vi "SettingButton_MenuSelect by Path.vi"(8 "error in (no error)":errorcluster caption="错误输入（无错误）", 9 "QName":string, 10 "MenuPath":string, 11 "PCM PanelSplit 输入":refnum<class "PCM PanelSplit.lvclass"> caption="DNL_LabVIEW Object in") -> (0 "error out":errorcluster caption="错误输出", 3 "PCM PanelSplit 输出":refnum<class "PCM PanelSplit.lvclass"> caption="DNL_LabVIEW Object out")   [LabVIEW 2016, in "PCM PanelSplit.lvclass"]
uses:
  PCM PanelSplit.lvclass
  Display Mode.ctl
  <vilib>/Analysis/4window.llb/windowTd.ctl
  PanelSplitToolkit/QueueManager.llb/Insert.vi
  <vilib>/Analysis/NI_AALPro.lvlib
panel:
  in  "window":T1=1 caption="窗" items=["Rectangle"=0, "Hanning"=1, "Hamming"=2, "Blackman-Harris"=3, "Exact Blackman"=4, "Blackman"=5, "Flat Top"=6, "4 Term B-Harris "=7, "7 Term B-Harris"=8, "Low Sidelobe"=9, "Blackman Nuttall"=11, "Triangle"=30, "Bartlett-Hanning"=31, "Bohman"=32, "Parzen"=33, "Welch"=34, "Kaiser"=60, "Dolph-Chebyshev"=61, "Gaussian"=62]
  in  "Display Mode":T2
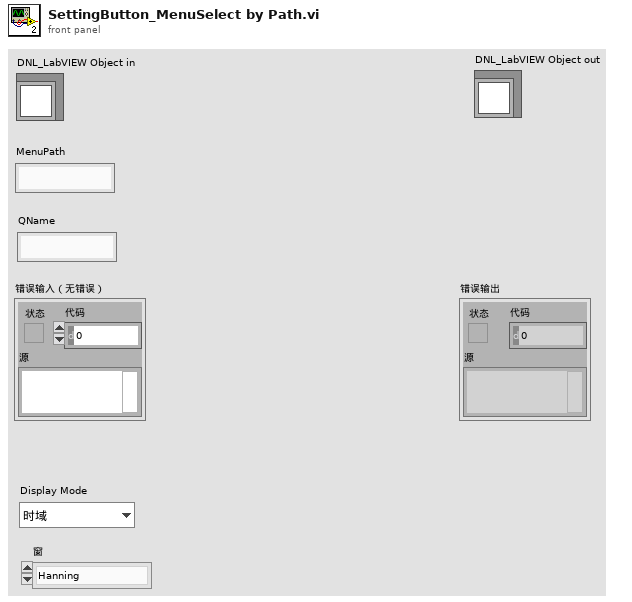
[diagram p1: front panel]
types:
  T1 = typedef "NI_AALPro.lvlib/windowTd.ctl" = u32
  T2 = typedef "PCM PanelSplit.lvclass/Display Mode.ctl" = enum16{"时域", "频谱", "功率谱"}
  T3 = typedef "PCM PanelSplit.lvclass/Display Config.ctl" = cluster{"Display Mode":T2, "ChTag[]":string[], "window":T1, "Range":T4}
  T4 = typedef "LVRangeTypeDef.ctl" = cluster{"Minimum":dbl, "Maximum":dbl, "Increment":dbl, "Minor Increment":dbl, "Start":dbl}
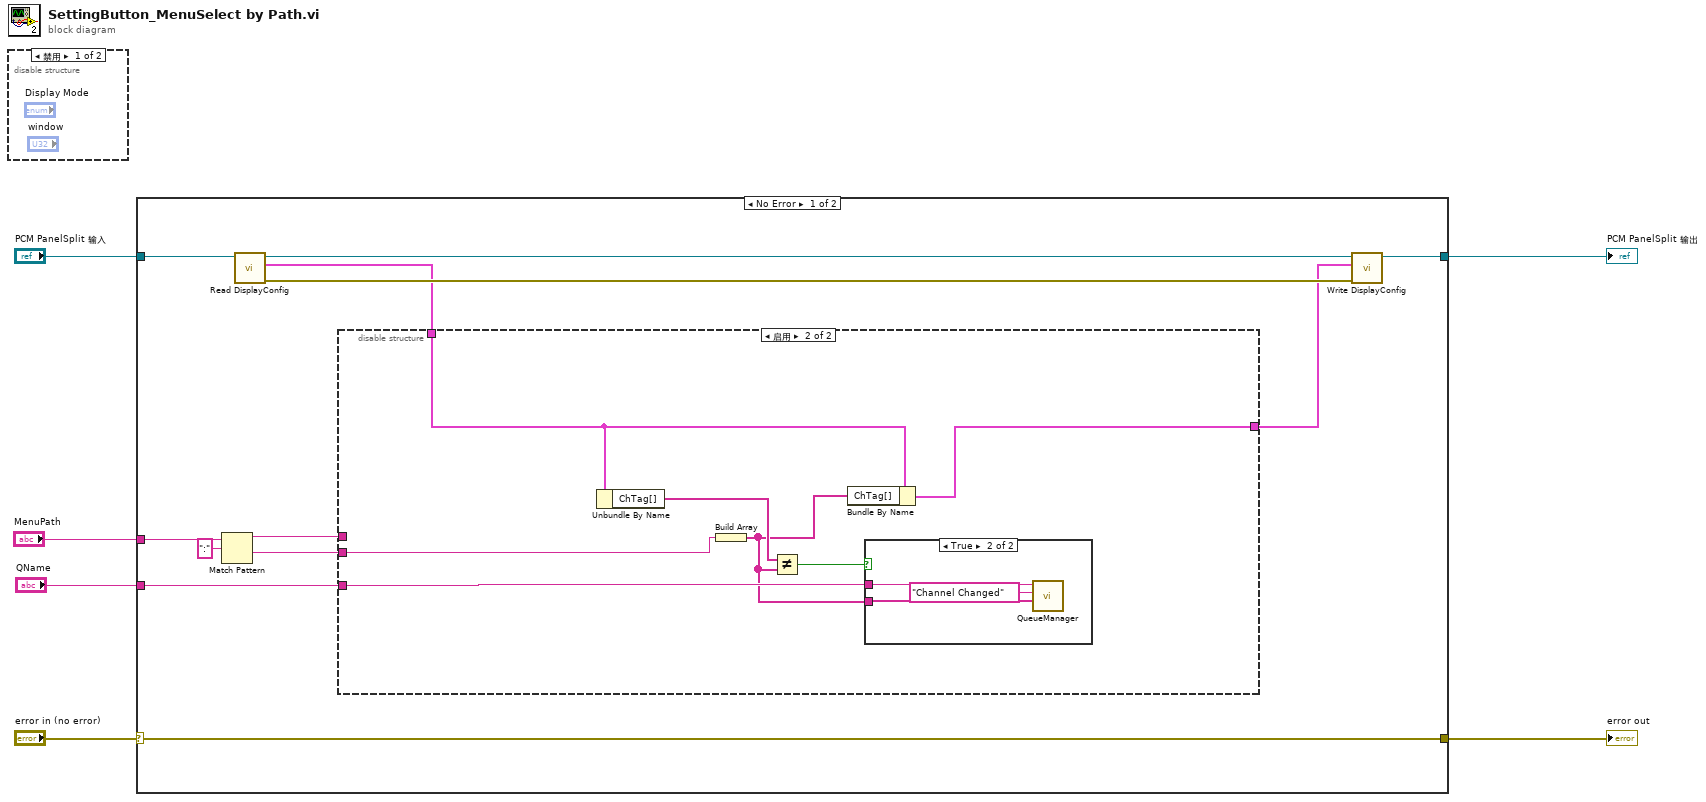
[diagram p0: block diagram]
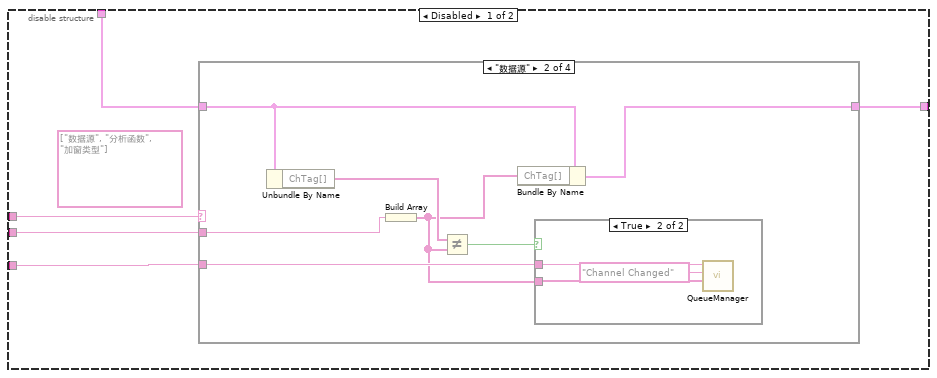
[diagram p3: hidden frame]
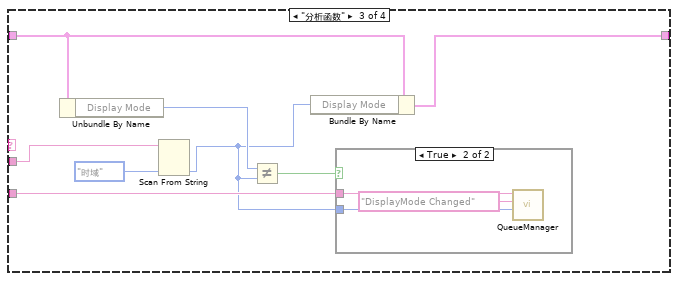
[diagram p6: hidden frame]
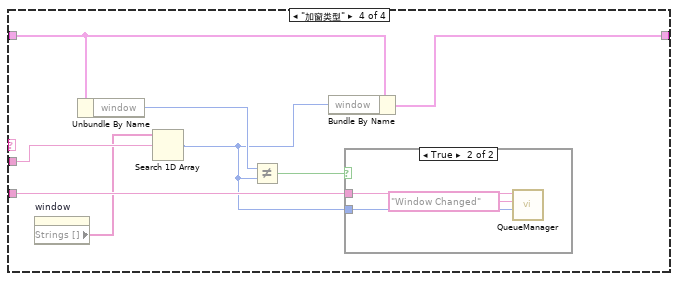
[diagram p8: hidden frame]
diagram:
  n1 = disable-structure shown="禁用" {
    frame Disabled {
    }
    frame Enabled {
    }
  }
  n2 = case shown="No Error" "error in (no error)" {
    selector: "error in (no error)" -> [w18 w68]
    tunnel: [w18 w68] -> w5
    tunnel: [w15 w67] -> w3
    tunnel: "PCM PanelSplit 输入" -> [w17 w67]
    tunnel: "MenuPath" -> [w13 _]
    tunnel: "QName" -> [w9 _]
    frame No Error {
      n3 = Match Pattern(string=w13, regular expression=":" ("正则表达式")) -> (before substring=w11:string, after substring=w7:string)  [unwired: 1 in, 2 out]
      n4 = call "Read DisplayConfig.vi"("PCM PanelSplit 输入"=w17) -> ("error out"=w14:errorcluster, "Display Config"=w10:T3, "PCM PanelSplit 输出"=w16:refnum<class "PCM PanelSplit.lvclass">)  [unwired: 8 in]
      n5 = disable-structure shown="启用" {
        disable-tunnel: w11 -> [w23 _]
        disable-tunnel: w10 -> [w22 w63]
        disable-tunnel: w9 -> [w21 w62]
        disable-tunnel: [w20 w61] -> w8
        disable-tunnel: w7 -> [w19 w60]
        frame Disabled {
          (unwired) string[] ["数据源", "分析函数", "加窗类型"] ("项名称")
          n6 = case shown="\"数据源\"" w23 {
            tunnel: w22 -> [w24 w28 w39 w50]
            tunnel: w21 -> [_ w29 w40 w51]
            tunnel: [w24 w27 w38 w49] -> w20
            tunnel: w19 -> [_ w25 w35 w47]
            frame "假", Default {
            }
            frame "数据源" {
              n7 = Unbundle By Name(w28) -> ("ChTag[]"=w31:string[])
              n8 = Build Array(w25) -> (w26:string[])
              n9 = Not Equal?(x=w31, y=w26) -> (x != y?=w30:bool)
              n10 = Bundle By Name(cluster=w28, "ChTag[]"=w26) -> (w27:T3)
              n11 = case shown="True" w30 {
                tunnel: w29 -> [_ w34]
                tunnel: w26 -> [_ w32]
                frame False {
                }
                frame True {
                  n12 = call-poly "QueueManager.vi"("Data"=w32, "Event"="Channel Changed", "QueueName"=w34) -> ()  [unwired: 7 in, 2 out]
                }
              }
            }
            frame "分析函数" {
              n13 = Unbundle By Name(w39) -> ("Display Mode"=w42:T2)
              n14 = Scan From String(input string=w35, default 1=Display_Mode."时域" ("Display Mode")) -> (output 1=w36:T2)  [unwired: 3 in, 3 out]
              n15 = Not Equal?(x=w42, y=w36) -> (x != y?=w41:bool)
              n16 = Bundle By Name(cluster=w39, "Display Mode"=w36) -> (w38:T3)
              n17 = case shown="True" w41 {
                tunnel: w40 -> [_ w45]
                tunnel: w36 -> [_ w43]
                frame False {
                }
                frame True {
                  n18 = call-poly "QueueManager.vi"("Data"=w43, "Event"="DisplayMode Changed", "QueueName"=w45) -> ()  [unwired: 7 in, 2 out]
                }
              }
            }
            frame "加窗类型" {
              n19 = property on="window" class="Ring (strict)"() -> ("Strings []"=w46:string[])  [unwired: 2 in, 2 out]
              n20 = Unbundle By Name(w50) -> ("window"=w53:T1)
              n21 = Search 1D Array(1D array=w46, element=w47) -> (index of element=w48:i32)  [unwired: 1 in]
              n22 = Not Equal?(x=w53, y=w48) -> (x != y?=w52:bool)
              n23 = Bundle By Name(cluster=w50, "window"=w48) -> (w49:T3)
              n24 = case shown="True" w52 {
                tunnel: w51 -> [_ w56]
                tunnel: w48 -> [_ w54]
                frame False {
                }
                frame True {
                  n25 = call-poly "QueueManager.vi"("Data"=w54, "Event"="Window Changed", "QueueName"=w56) -> ()  [unwired: 7 in, 2 out]
                }
              }
            }
          }
        }
        frame Enabled {
          n26 = Unbundle By Name(w63) -> ("ChTag[]"=w59:string[])
          n27 = Build Array(w60) -> (w57:string[])
          n28 = Not Equal?(x=w59, y=w57) -> (x != y?=w58:bool)
          n29 = Bundle By Name(cluster=w63, "ChTag[]"=w57) -> (w61:T3)
          n30 = case shown="True" w58 {
            tunnel: w62 -> [_ w66]
            tunnel: w57 -> [_ w64]
            frame False {
            }
            frame True {
              n31 = call-poly "QueueManager.vi"("Data"=w64, "Event"="Channel Changed", "QueueName"=w66) -> ()  [unwired: 7 in, 2 out]
            }
          }
        }
      }
      n32 = call "Write DisplayConfig.vi"("error in"=w14, "Display Config"=w8, "PCM PanelSplit 输入"=w16) -> ("PCM PanelSplit 输出"=w15:refnum<class "PCM PanelSplit.lvclass">)  [unwired: 7 in, 1 out]
    }
    frame Error {
    }
  }
  "error out" <- w5
  "PCM PanelSplit 输出" <- w3
